vi "provide_note_book_info.vi"(8 "error in (no error)":errorcluster, 10 "notebook string in":string, 11 "DataCollectionMG091001IntrinsicImaging in":refnum<class "DataCollectionMG091001IntrinsicImaging.lvclass">) -> (0 "error out":errorcluster, 2 "notebook string out":string, 3 "DataCollectionMG091001IntrinsicImaging out":refnum<class "DataCollectionMG091001IntrinsicImaging.lvclass">)   [LabVIEW 2010, in "DataCollectionMG091001IntrinsicImaging.lvclass"]
uses:
  DataCollectionMG091001IntrinsicImaging.lvclass
  DataCollectionDL091104Scaffold/DataCollectionDL091104Scaffold/DataCollectionDL091104Scaffold.lvclass
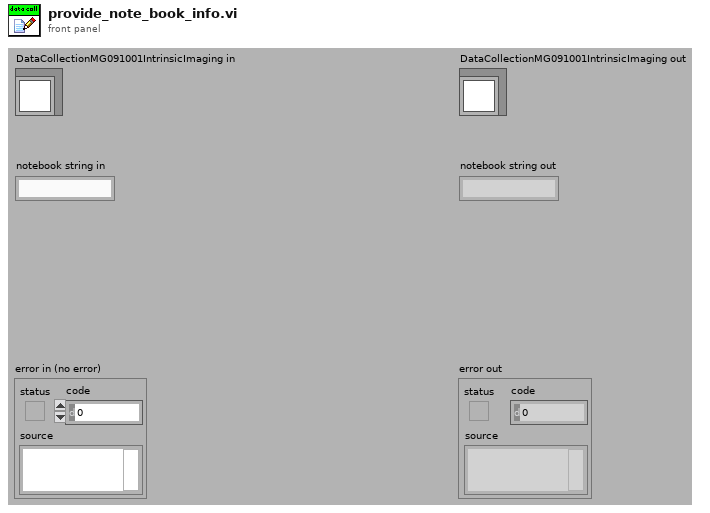
[diagram p1: front panel]
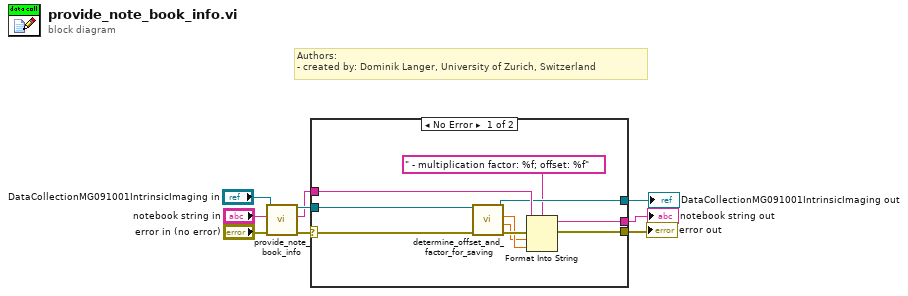
[diagram p0: block diagram]
diagram:
  # "Authors: \n- created by: Dominik Langer, University of Zurich, Switzerland"
  n1 = call-parent "provide_note_book_info.vi"("error in (no error)"="error in (no error)", "notebook string in"="notebook string in", "DataCollectionDL091104Scaffold in"="DataCollectionMG091001IntrinsicImaging in") -> ("error out"=w6:errorcluster, "notebook string out"=w4:string, "DataCollectionDL091104Scaffold out"=w5:refnum<class "DataCollectionMG091001IntrinsicImaging.lvclass">)  [unwired: 6 in]
  n2 = case shown="No Error" w6 {
    selector: w6 -> [w19 w20]
    tunnel: w5 -> [w18 w22]
    tunnel: w4 -> [w16 w21]
    tunnel: [w15 w21] -> w3
    tunnel: [w14 w20] -> w2
    tunnel: [w13 w22] -> w1
    frame No Error {
      n3 = call-dynamic "determine_offset_and_factor_for_saving.vi"("error in (no error)"=w19, "DataCollectionMG091001IntrinsicImaging in"=w18) -> ("error out"=w17:errorcluster, "factor"=w10:dbl, "offset"=w11:dbl, "DataCollectionMG091001IntrinsicImaging out"=w13:refnum<class "DataCollectionMG091001IntrinsicImaging.lvclass">)  [unwired: 6 in]
      n4 = Format Into String(format string=" - multiplication factor: %f; offset: %f", initial string=w16, error in=w17, w10, w11) -> (resulting string=w15:string, error out=w14:errorcluster)
    }
    frame Error {
    }
  }
  "error out" <- w2
  "DataCollectionMG091001IntrinsicImaging out" <- w1
  "notebook string out" <- w3
